vi "SpectrumCursor_init.vi"(0 "MapFunction":T1 items=["Total"=0, "Peak"=4, "Area"=2, "Value"=1, "Ratio"=3], 2 "Spectrum":refnum<vi>) -> ()   [LabVIEW 2010]
uses:
  _TypeDefs/MapFunctions.ctl
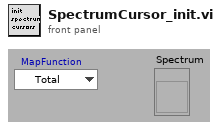
[diagram p1: front panel]
types:
  T1 = typedef "MapFunctions.ctl" = u16
  T2 = cluster{"Name":string, "Color":u32, "Style":u8, "Point Style":u8, "Name Visible":bool, "Allow Drag":bool, "Cursor Mode":u32, "Plot":i32, "Index":i32, "Position":cluster{"X":dbl, "Y":dbl}, "X Scale":u32, "Y Scale":u32, "Watch Plots":i32[], "Watch All Plots":bool, "Plot Area":i32, "Label Offset":cluster{"X":dbl, "Y":dbl}}[]
  T3 = cluster{"Name":string, "Color":u32, "Style":u8, "Point Style":u8, "Name Visible":bool, "Allow Drag":bool, "Cursor Mode":u32, "Plot":i32, "Index":i32, "Position":cluster{"X":dbl, "Y":dbl}, "X Scale":u32, "Y Scale":u32, "Watch Plots":i32[], "Watch All Plots":bool, "Plot Area":i32, "Label Offset":cluster{"X":dbl, "Y":dbl}}
  T4 = typedef "LVCursorListTypeDef.ctl" = cluster{"Name":string, "Color":u32, "Style":u8, "Point Style":u8, "Name Visible":bool, "Allow Drag":bool, "Cursor Mode":u32, "Plot":i32, "Index":i32, "Position":cluster{"X":dbl, "Y":dbl}, "X Scale":u32, "Y Scale":u32, "Watch Plots":i32[], "Watch All Plots":bool, "Plot Area":i32, "Label Offset":cluster{"X":dbl, "Y":dbl}}[]
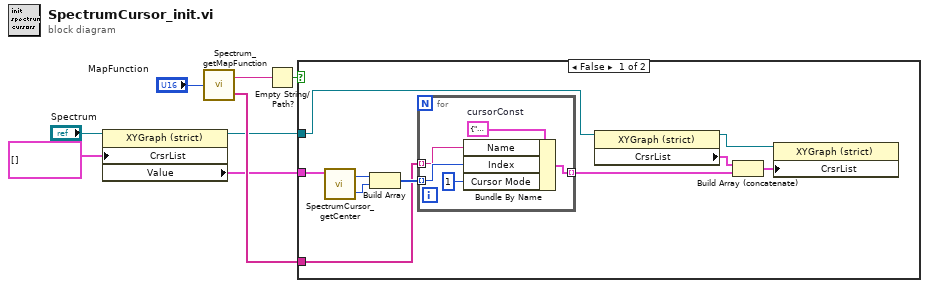
[diagram p0: block diagram]
diagram:
  n1 = property on="Eigenschaftsknoten" class="XYGraph (strict)"(reference="Spectrum", "CrsrList"=T2 [] ("Cursor List")) -> (reference out=w2:refnum<vi>, "Value"=w1:cluster{dbl[], dbl[]})  [unwired: 1 in, 1 out]
  n2 = call "Spectrum_getMapFunction.vi"("MapFunction"="MapFunction") -> ("CursorNames"=w6:string[], "Function"=w5:string)
  n3 = Empty String/Path?(string/path=w5) -> (empty?=w8:bool)
  n4 = case shown="False" w8 {
    tunnel: w6 -> [w12 _]
    tunnel: w2 -> [w11 _]
    tunnel: w1 -> [w9 _]
    frame False {
      n5 = call "SpectrumCursor_getCenter.vi"("Value"=w9) -> ("cursor2X"=w15:i64, "cursor1X"=w14:i64)  [unwired: 3 in]
      n6 = Build Array(w14, w15) -> (w16:i64[])
      n7 = for {
        tunnel: w12 -> [w22] mode=indexing
        tunnel: w16 -> [w23] mode=indexing
        tunnel: [w20] -> w13 mode=indexing
        w21 = T3 {"Name"="cursor", "Color"=1985280, "Style"=2, "Point Style"=6, "Name Visible"=FALSE, "Allow Drag"=TRUE, "Cursor Mode"=0, "Plot"=0, "Index"=0, "Position"={"X"=0.0, "Y"=0.0}, "X Scale"=0, "Y Scale"=0, "Watch Plots"=[], "Watch All Plots"=FALSE, "Plot Area"=0, "Label Offset"={"X"=0.0, "Y"=0.0}}  # cursorConst
        n8 = Bundle By Name(cluster=w21, "Name"=w22, "Index"=w23, "Cursor Mode"=u32 1) -> (w20:T3)
      }
      n9 = property on="Eigenschaftsknoten" class="XYGraph (strict)"(reference=w11) -> (reference out=w10:refnum<vi>, "CrsrList"=w18:T4)  [unwired: 1 in, 1 out]
      n10 = Build Array (concatenate)(w18, w13) -> (w17:T4)
      n11 = property on="Eigenschaftsknoten" class="XYGraph (strict)"(reference=w10, "CrsrList"=w17) -> ()  [unwired: 1 in, 2 out]
    }
    frame True {
    }
  }
